vi "Get Channel Connection.vi"(8 "error in (no error)":errorcluster, 9 "Connection Type":string, 10 "Channel":string, 11 "2010 Connection Lookup in":refnum<class "2010 Connection Lookup.lvclass">) -> (0 "error out":errorcluster, 2 "Connected Channel":string, 3 "2010 Connection Lookup out":refnum<class "2010 Connection Lookup.lvclass">)   [LabVIEW 2020, in "Routing Templates.lvlib" / "2010 Connection Lookup.lvclass"]
uses:
  2010 Connection Lookup.lvclass
  SLSC-2010 Channels.ctl
  SLSC-2010 Connection Type.ctl
  <vilib>/Utility/error.llb/Error Cluster From Error Code.vi
  <vilib>/regexp/Match Regular Expression.xnode
  <vilib>/ErrorRing/Error Ring.xnode
  2010 Connection Lookup.lvclass/2010 Connection Lookup.ctl
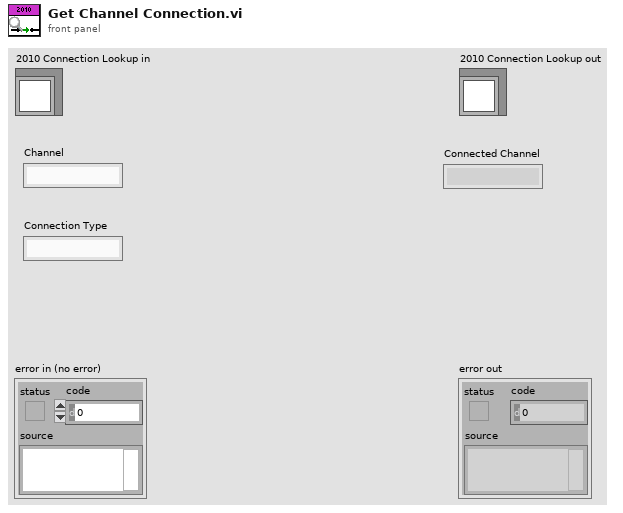
[diagram p1: front panel]
types:
  T1 = typedef "Routing Templates.lvlib/2010 Connection Lookup.lvclass/SLSC-2010 Connection Type.ctl" = enum16{"<INVALID>", "Disconnected", "Passthrough", "Real-Sim", "Short Pair", "Fault A", "Fault B", "Fault C", "Fault D"}
  T2 = typedef "Routing Templates.lvlib/2010 Connection Lookup.lvclass/SLSC-2010 Channels.ctl" = enum16{"<INVALID>", "J1Ch0p", "J1Ch0n", "J1Ch1p", "J1Ch1n", "J1Ch2p", "J1Ch2n", "J1Ch3p", "J1Ch3n", "J1Ch4p", "J1Ch4n", "J1Ch5p", "J1Ch5n", "J1Ch6p", "J1Ch6n", "J1Ch7p", "J1Ch7n", "J1Ch8p", "J1Ch8n", "J1Ch9p", "J1Ch9n", "J1Ch10p", "J1Ch10n", "J1Ch11p", "J1Ch11n", "J1Ch12p", "J1Ch12n", "J1Ch13p", "J1Ch13n", "J1Ch14p", "J1Ch14n", "J1Ch15p", "J1Ch15n", "J2Ch16p", "J2Ch16n", "J2Ch17p", "J2Ch17n", "J2Ch18p", "J2Ch18n", "J2Ch19p", "J2Ch19n", "J2Ch20p", "J2Ch20n", "J2Ch21p", "J2Ch21n", "J2Ch22p", "J2Ch22n", "J2Ch23p", "J2Ch23n", "J2Ch24p", "J2Ch24n", "J2Ch25p", "J2Ch25n", "J2Ch26p", "J2Ch26n", "J2Ch27p", "J2Ch27n", "J2Ch28p", "J2Ch28n", "J2Ch29p", "J2Ch29n", "J2Ch30p", "J2Ch30n", "J2Ch31p", "J2Ch31n"}
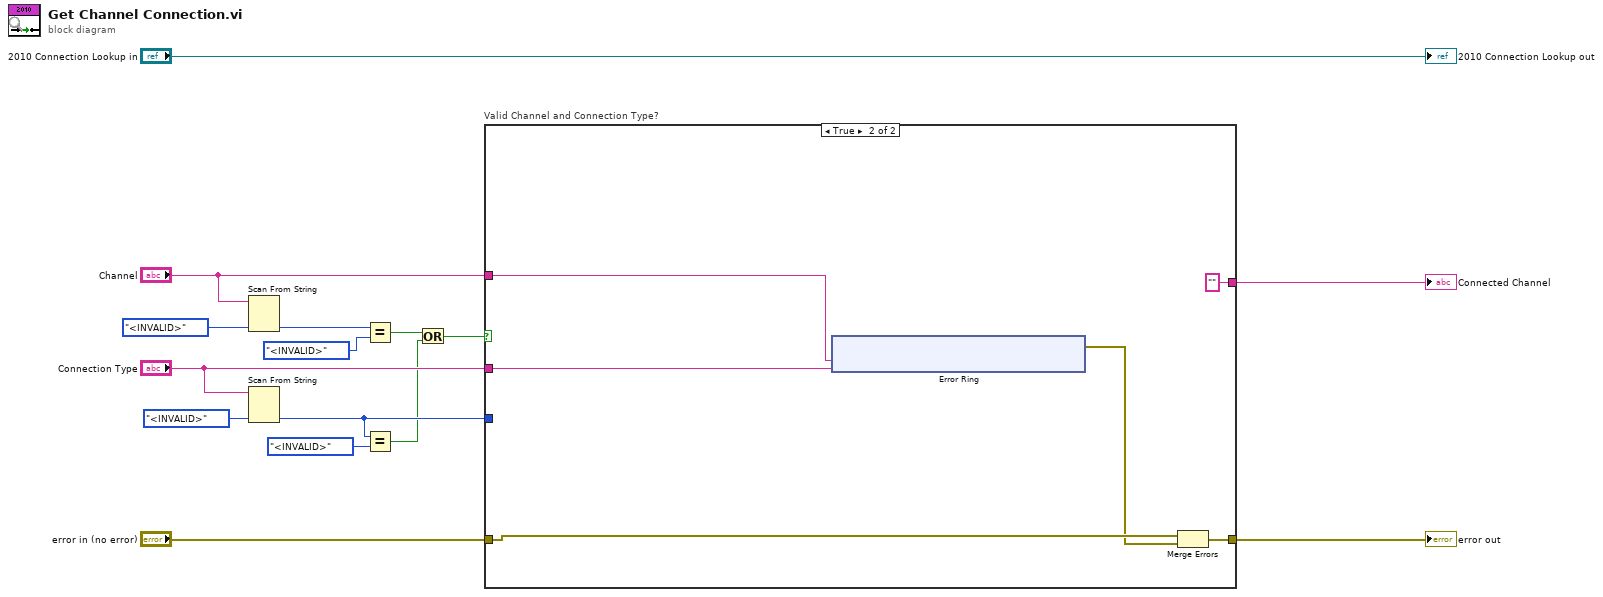
[diagram p0: block diagram]
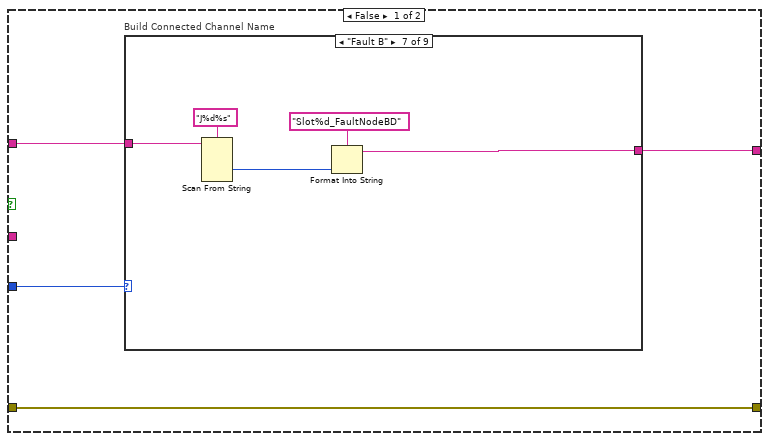
[diagram p2: hidden frame]
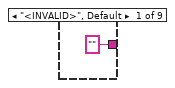
[diagram p3: hidden frame]
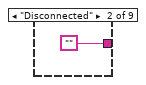
[diagram p4: hidden frame]
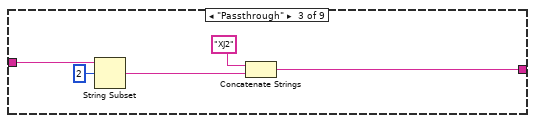
[diagram p5: hidden frame]
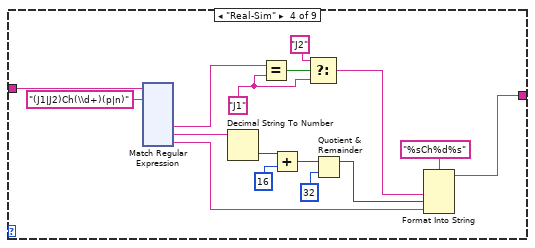
[diagram p6: hidden frame]
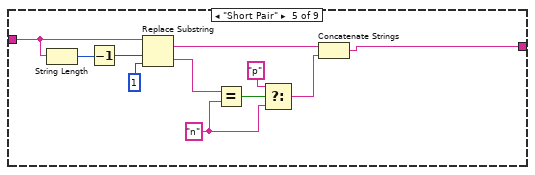
[diagram p7: hidden frame]
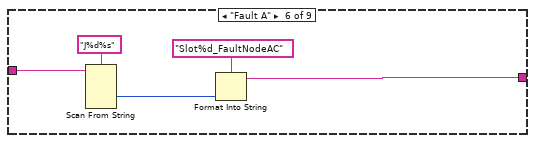
[diagram p8: hidden frame]
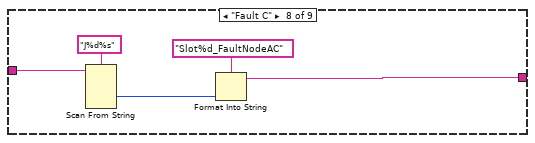
[diagram p9: hidden frame]
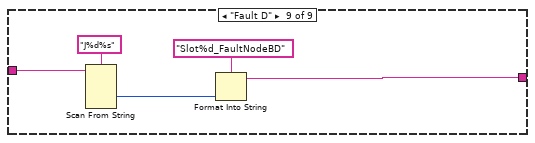
[diagram p10: hidden frame]
diagram:
  n1 = Scan From String(input string="Channel", default 1=SLSC-2010_Channels."<INVALID>" ("SLSC-2010 Channels")) -> (output 1=w7:T2)  [unwired: 3 in, 3 out]
  n2 = Scan From String(input string="Connection Type", default 1=SLSC-2010_Connection_Type."<INVALID>" ("Connnection Type")) -> (output 1=w5:T1)  [unwired: 3 in, 3 out]
  n3 = Equal?(x=w7, y=SLSC-2010_Channels."<INVALID>" ("SLSC-2010 Channels")) -> (x = y?=w3:bool)
  n4 = Equal?(x=w5, y=SLSC-2010_Connection_Type."<INVALID>") -> (x = y?=w2:bool)
  n5 = Or(x=w3, y=w2) -> (x .or. y?=w1:bool)
  n6 = case "Valid Channel and Connection Type?" shown="True" w1 {
    tunnel: [w19 ""] -> w14
    tunnel: w5 -> [w18 _]
    tunnel: "Channel" -> [w17 w197]
    tunnel: [w16 w194] -> w10
    tunnel: "error in (no error)" -> [w16 w193]
    tunnel: "Connection Type" -> [_ w196]
    frame False {
      n7 = case "Build Connected Channel Name" shown="\"Fault B\"" w18 {
        tunnel: w17 -> [_ _ w26 w42 w170 w176 w181 w186 w191]
        tunnel: ["" "" w22 w28 w161 w172 w177 w182 w187] -> w19
        frame "<INVALID>", Default {
        }
        frame "Disconnected" {
        }
        frame "Passthrough" {
          n8 = String Subset(string=w26, offset (0)=2) -> (substring=w24:string)  [unwired: 1 in]
          n9 = Concatenate Strings("XJ2" ("string"), w24) -> (w22:string)
        }
        frame "Real-Sim" {
          w38 = "J1" ("y")
          n10 = xnode "Match Regular Expression"("input string"=w42, "regular expression"="(J1|J2)Ch(\\d+)(p|n)") -> ("submatch 1"=w40:string, "submatch 2"=w36:string, "submatch 3"=w27:string)  [unwired: 4 in, 5 out]
          n11 = Decimal String To Number(string=w36) -> (number=w35:i32)  [unwired: 2 in, 1 out]
          n12 = Equal?(x=w40, y=w38) -> (x = y?=w39:bool)
          n13 = Add(x=w35, y=16) -> (x+y=w33:i32)
          n14 = Select(t="J2" ("y"), s=w39, f=w38) -> (s? t:f=w30:string)
          n15 = Quotient & Remainder(x=w33, y=32) -> (x-y*floor(x/y)=w29:i32)  [unwired: 1 out]
          n16 = Format Into String(format string="%sCh%d%s", w30, w29, w27) -> (resulting string=w28:string)  [unwired: 2 in, 1 out]
        }
        frame "Short Pair" {
          w167 = "n" ("y")
          n17 = String Length(string=w170) -> (length=w169:i32)
          n18 = Decrement(x=w169) -> (x-1=w168:i32)
          n19 = Replace Substring(2:1 ("length (len. of substring)"), 3:w168, 5:w170) -> (0:w164:string, 1:w163:string)  [unwired: 1 in]
          n20 = Equal?(x=w164, y=w167) -> (x = y?=w166:bool)
          n21 = Select(t="p" ("y"), s=w166, f=w167) -> (s? t:f=w162:string)
          n22 = Concatenate Strings(w163, w162) -> (w161:string)
        }
        frame "Fault A" {
          n23 = Scan From String(format string="J%d%s", input string=w176) -> (output 1=w174:i32)  [unwired: 5 in, 3 out]
          n24 = Format Into String(format string="Slot%d_FaultNodeAC", w174) -> (resulting string=w172:string)  [unwired: 2 in, 1 out]
        }
        frame "Fault B" {
          n25 = Scan From String(format string="J%d%s", input string=w181) -> (output 1=w179:i32)  [unwired: 5 in, 3 out]
          n26 = Format Into String(format string="Slot%d_FaultNodeBD", w179) -> (resulting string=w177:string)  [unwired: 2 in, 1 out]
        }
        frame "Fault C" {
          n27 = Scan From String(format string="J%d%s", input string=w186) -> (output 1=w184:i32)  [unwired: 5 in, 3 out]
          n28 = Format Into String(format string="Slot%d_FaultNodeAC", w184) -> (resulting string=w182:string)  [unwired: 2 in, 1 out]
        }
        frame "Fault D" {
          n29 = Scan From String(format string="J%d%s", input string=w191) -> (output 1=w189:i32)  [unwired: 5 in, 3 out]
          n30 = Format Into String(format string="Slot%d_FaultNodeBD", w189) -> (resulting string=w187:string)  [unwired: 2 in, 1 out]
        }
      }
    }
    frame True {
      n31 = xnode "Error Ring"("parameter 0"=w197, "parameter 1"=w196) -> ("error out"=w192:errorcluster)
      n32 = Merge Errors(w193, w192) -> (w194:errorcluster)
    }
  }
  "error out" <- w10
  "Connected Channel" <- w14
  "2010 Connection Lookup out" <- "2010 Connection Lookup in"
